vi "ControlCamera.vi"(0 "NumX":i16=640, 1 "StartX":i16=1, 3 "Mode":u16(ring)=4 items=["Exposition guideur"=0, "Guidage"=2, "Piedestal"=3, "Exposition simple"=4, "Mode continu"=5, "Calibration"=8], 4 "ExpTime":dbl, 5 "BinX":i16=1, 6 "N-images(obsolete)":i32, 7 "MaxIm.ICCDCamera":refnum<k7>, 9 "BinY":i16=1, 11 "NumY":i16=480, 12 "StartY":i16=1, 14 "DEC":i16) -> (8 "Done":bool, 10 "ICCDError":errorcluster, 15 "GuiderArrayError":errorcluster)   [LabVIEW 2011]
uses:
  Globals.vi
panel:
  in  "RemoveDark":bool
  out "NumXout":i16=657
  out "NumYout":i16=495
  out "DarkImg":i32[][](array[numeric])
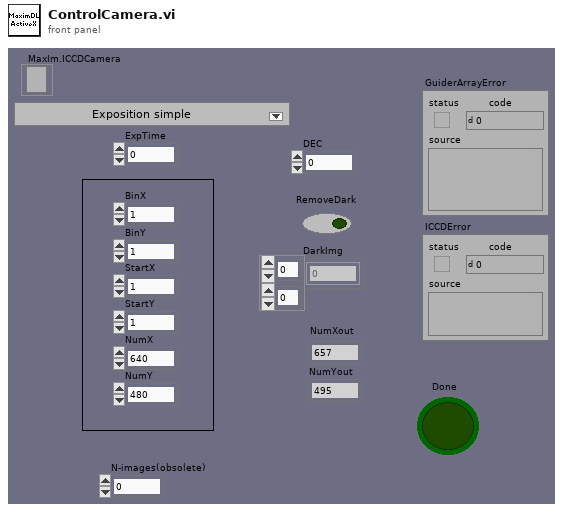
[diagram p1: front panel]
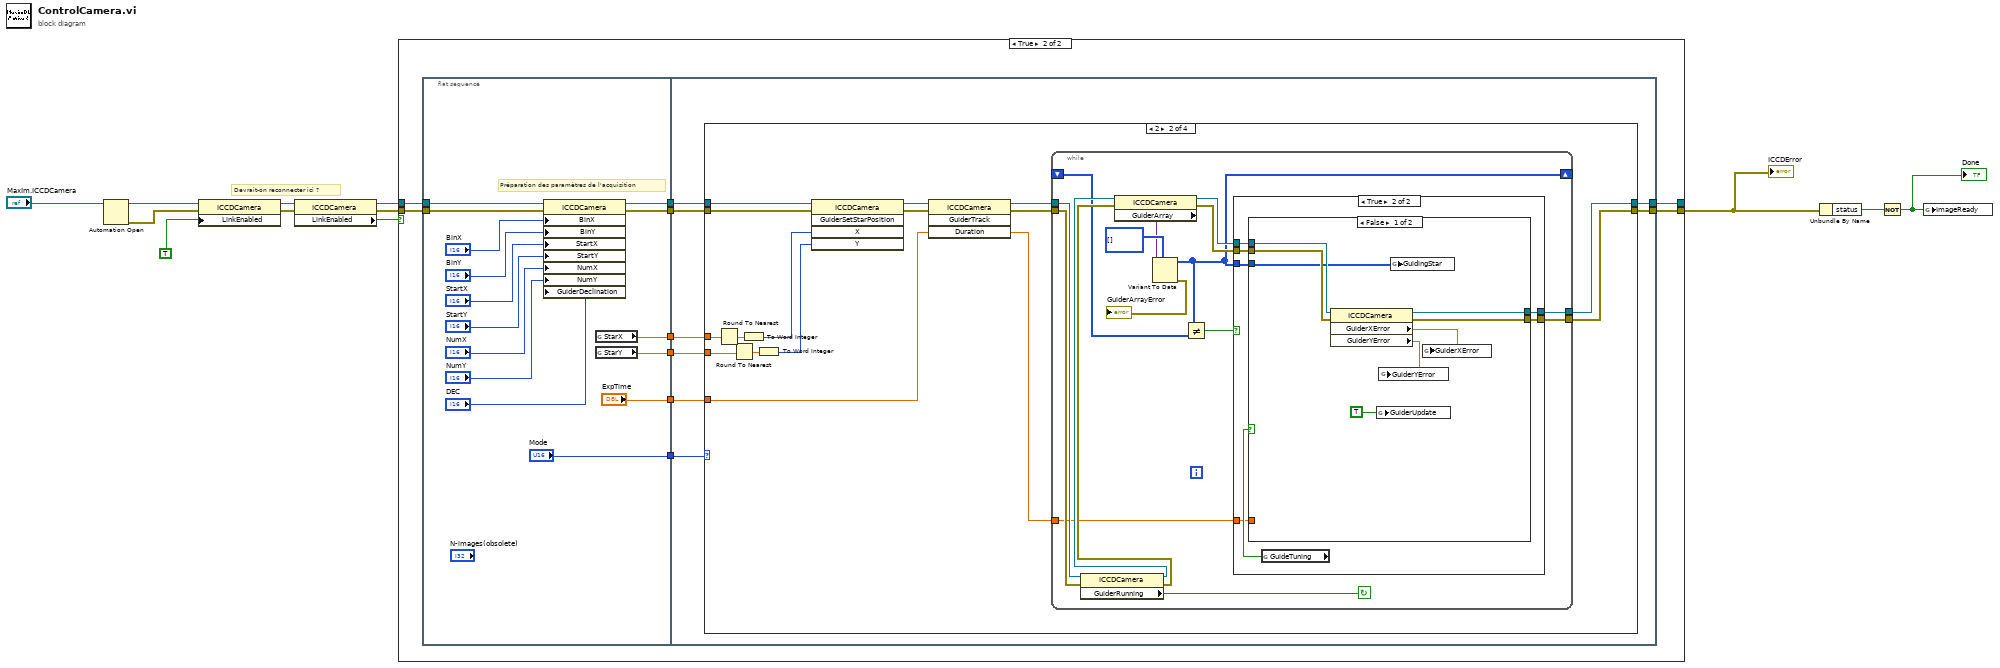
[diagram p0: block diagram]
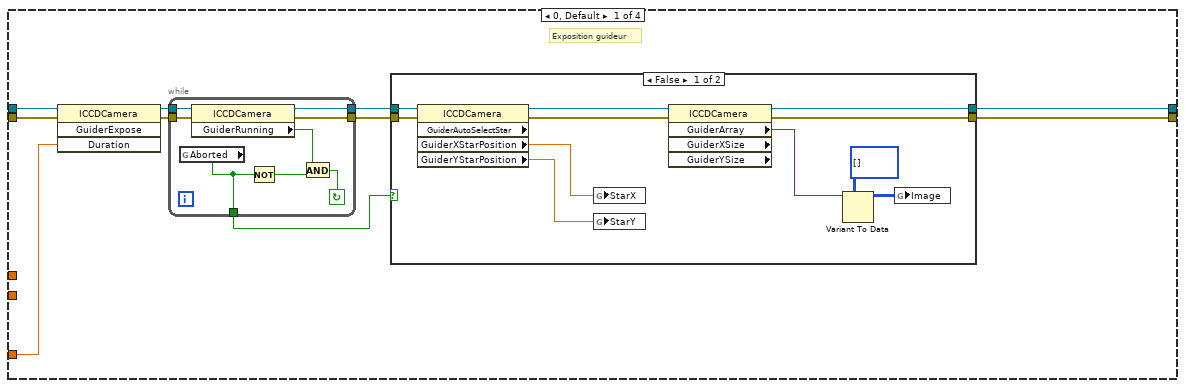
[diagram p3: hidden frame]
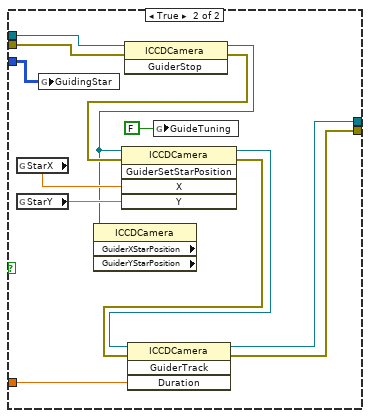
[diagram p6: hidden frame]
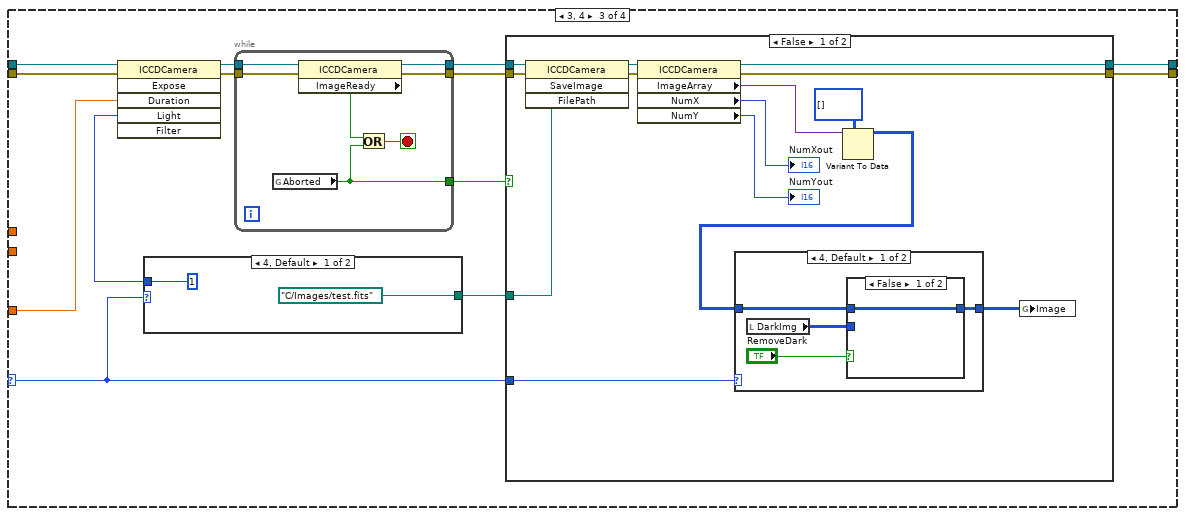
[diagram p7: hidden frame]
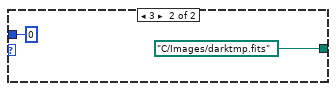
[diagram p8: hidden frame]
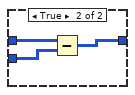
[diagram p9: hidden frame]
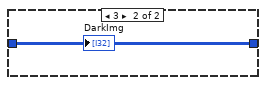
[diagram p10: hidden frame]
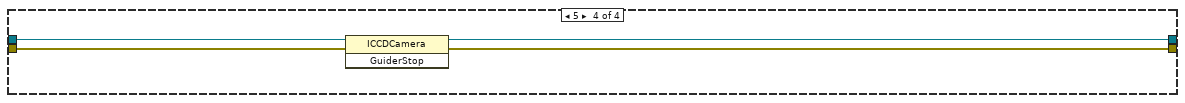
[diagram p12: hidden frame]
diagram:
  # "Devrait-on reconnecter ici ?"
  n1 = Automation Open(Automation Refnum="MaxIm.ICCDCamera") -> (Automation Refnum=w4:refnum<k7>, error out=w3:errorcluster)  [unwired: 3 in]
  n2 = property class="ICCDCamera"(reference=w4, error in=w3, "LinkEnabled"=TRUE) -> (reference out=w6:refnum<k7>, error out=w5:errorcluster)
  n3 = property class="ICCDCamera"(reference=w6, error in=w5) -> (reference out=w10:refnum<k7>, error out=w9:errorcluster, "LinkEnabled"=w11:bool)
  n4 = case shown="True" w11 {
    tunnel: w10 -> [w13 w24]
    tunnel: w9 -> [w14 w22]
    tunnel: [w14 w18] -> w1
    tunnel: [w13 w17] -> _
    frame False {
    }
    frame True {
      n5 = flat-sequence {
        tunnel: w24 -> [w39]
        tunnel: [w38] -> w23
        tunnel: w22 -> [w37]
        tunnel: [w36] -> w21
        tunnel: ["ExpTime"] -> w20
        tunnel: ["Mode"] -> w19
        tunnel: [w27] -> w16
        tunnel: [w26] -> w15
        tunnel: w23 -> [w47]
        tunnel: w21 -> [w46]
        tunnel: w20 -> [w45]
        tunnel: [w44] -> w17
        tunnel: [w43] -> w18
        tunnel: w19 -> [w42]
        tunnel: w16 -> [w41]
        tunnel: w15 -> [w40]
        frame #0 {
          # "Préparation des paramètres de l'acquisition"
          n6 = property class="ICCDCamera"(reference=w39, error in=w37, "BinX"="BinX", "BinY"="BinY", "StartX"="StartX", "StartY"="StartY", "NumX"="NumX", "NumY"="NumY", "GuiderDeclination"="DEC") -> (reference out=w38:refnum<k7>, error out=w36:errorcluster)
          n7 = global read "Globals.vi" "StarX"() -> (w27:sgl)
          n8 = global read "Globals.vi" "StarY"() -> (w26:sgl)
        }
        frame #1 {
          n9 = case shown="2" w42 {
            selector: w42 -> [_ _ w143 _]
            tunnel: w47 -> [w53 w94 w147 w193]
            tunnel: w46 -> [w52 w93 w146 w192]
            tunnel: w45 -> [w51 w84 w148 _]
            tunnel: [w49 w81 w144 w191] -> w44
            tunnel: [w48 w80 w145 w190] -> w43
            tunnel: w41 -> [_ w92 _ _]
            tunnel: w40 -> [_ w88 _ _]
            frame 0, Default {
              # "Exposition guideur"
              n10 = invoke class="ICCDCamera" method="GuiderExpose"(reference=w53, error in=w52, "Duration"=w51) -> (reference out=w57:refnum<k7>, error out=w55:errorcluster)  [unwired: 1 in, 2 out]
              n11 = while {
                tunnel: [w75] -> w54
                tunnel: w55 -> [w76]
                tunnel: [w77] -> w56
                tunnel: w57 -> [w78]
                tunnel: [w71] -> w50
                stop <- w74 continue-if-true
                n12 = global read "Globals.vi" "Aborted"() -> (w71:bool)
                n13 = property class="ICCDCamera"(reference=w78, error in=w76) -> (reference out=w77:refnum<k7>, error out=w75:errorcluster, "GuiderRunning"=w73:bool)
                n14 = Not(x=w71) -> (.not. x?=w72:bool)
                n15 = And(x=w73, y=w72) -> (x .and. y?=w74:bool)
              }
              n16 = case shown="False" w50 {
                tunnel: w56 -> [w68 w70]
                tunnel: w54 -> [w67 w69]
                tunnel: [w59 w70] -> w49
                tunnel: [w58 w69] -> w48
                frame False {
                  n17 = property class="ICCDCamera" props=["GuiderAutoSelectStar", "GuiderXStarPosition", "GuiderYStarPosition"](reference=w68, error in=w67) -> (reference out=w66:refnum<k7>, error out=w60:errorcluster, "GuiderXStarPosition"=w62:sgl, "GuiderYStarPosition"=w61:sgl)  [unwired: 1 out]
                  n18 = global write "Globals.vi" "StarX"(w62) -> ()
                  n19 = global write "Globals.vi" "StarY"(w61) -> ()
                  n20 = property class="ICCDCamera" props=["GuiderArray", "GuiderXSize", "GuiderYSize"](reference=w66, error in=w60) -> (reference out=w59:refnum<k7>, error out=w58:errorcluster, "GuiderArray"=w65:variant)  [unwired: 2 out]
                  n21 = Variant To Data(type=i32[][] [], Variant=w65) -> (data=w63:i32[][])  [unwired: 1 in, 1 out]
                  n22 = global write "Globals.vi" "Image"(w63) -> ()
                }
                frame True {
                }
              }
            }
            frame 2 {
              n23 = Round To Nearest(number=w92) -> (nearest integer value=w91:sgl)
              n24 = Round To Nearest(number=w88) -> (nearest integer value=w89:sgl)
              n25 = To Word Integer(number=w91) -> (16bit integer=w90:i16)
              n26 = To Word Integer(number=w89) -> (16bit integer=w87:i16)
              n27 = invoke class="ICCDCamera" method="GuiderSetStarPosition"(reference=w94, error in=w93, "X"=w90, "Y"=w87) -> (reference out=w86:refnum<k7>, error out=w85:errorcluster)  [unwired: 1 in, 3 out]
              n28 = invoke class="ICCDCamera" method="GuiderTrack"(reference=w86, error in=w85, "Duration"=w84) -> (reference out=w83:refnum<k7>, error out=w82:errorcluster, "Duration"=w79:dbl)  [unwired: 1 in, 1 out]
              n29 = while {
                tunnel: [w108] -> w80
                tunnel: w82 -> [w109]
                tunnel: w83 -> [w110]
                shift-right: [w97] -> _
                shift-left: _ -> [w99]
                tunnel: [w96] -> w81
                tunnel: w79 -> [w95]
                stop <- w107 continue-if-true
                n30 = property class="ICCDCamera"(reference=w110, error in=w109) -> (reference out=w104:refnum<k7>, error out=w103:errorcluster, "GuiderRunning"=w107:bool)
                n31 = property class="ICCDCamera"(reference=w104, error in=w103) -> (reference out=w105:refnum<k7>, error out=w106:errorcluster, "GuiderArray"=w100:variant)
                n32 = Variant To Data(type=i16[][] [], Variant=w100) -> (data=w97:i16[][], error out=→"GuiderArrayError":errorcluster)  [unwired: 1 in]
                n33 = Not Equal?(x=w97, y=w99) -> (x != y?=w101:bool)
                n34 = case shown="True" w101 {
                  tunnel: w106 -> [w112 w117]
                  tunnel: w105 -> [w111 w118]
                  tunnel: [w112 w119] -> w108
                  tunnel: w97 -> [_ w116]
                  tunnel: [w111 w114] -> w96
                  tunnel: w95 -> [_ w113]
                  frame False {
                  }
                  frame True {
                    n35 = global read "Globals.vi" "GuideTuning"() -> (w115:bool)
                    n36 = case shown="False" w115 {
                      tunnel: [w127 w138] -> w119
                      tunnel: w118 -> [w123 w140]
                      tunnel: w117 -> [w122 w139]
                      tunnel: w116 -> [w121 w136]
                      tunnel: [w120 w129] -> w114
                      tunnel: w113 -> [_ w128]
                      frame False {
                        n37 = property class="ICCDCamera"(reference=w123, error in=w122) -> (reference out=w120:refnum<k7>, error out=w127:errorcluster, "GuiderXError"=w126:sgl, "GuiderYError"=w125:sgl)
                        n38 = global write "Globals.vi" "GuiderUpdate"(TRUE ("GuiderUpdate")) -> ()
                        n39 = global write "Globals.vi" "GuiderYError"(w125) -> ()
                        n40 = global write "Globals.vi" "GuidingStar"(w121) -> ()
                        n41 = global write "Globals.vi" "GuiderXError"(w126) -> ()
                      }
                      frame True {
                        n42 = global read "Globals.vi" "StarX"() -> (w132:sgl)
                        n43 = global read "Globals.vi" "StarY"() -> (w131:sgl)
                        n44 = global write "Globals.vi" "GuidingStar"(w136) -> ()
                        n45 = invoke class="ICCDCamera" method="GuiderStop"(reference=w140, error in=w139) -> (reference out=w130:refnum<k7>, error out=w135:errorcluster)  [unwired: 1 in, 1 out]
                        n46 = property class="ICCDCamera" props=["GuiderXStarPosition", "GuiderYStarPosition"](reference=w130) -> ()  [unwired: 1 in, 4 out]
                        n47 = invoke class="ICCDCamera" method="GuiderSetStarPosition"(reference=w130, error in=w135, "X"=w132, "Y"=w131) -> (reference out=w134:refnum<k7>, error out=w133:errorcluster)  [unwired: 1 in, 3 out]
                        n48 = invoke class="ICCDCamera" method="GuiderTrack"(reference=w134, error in=w133, "Duration"=w128) -> (reference out=w129:refnum<k7>, error out=w138:errorcluster)  [unwired: 1 in, 2 out]
                        n49 = global write "Globals.vi" "GuideTuning"(FALSE) -> ()
                      }
                    }
                  }
                }
              }
            }
            frame 3, 4 {
              n50 = case shown="4, Default" w143 {
                tunnel: [path "C:/Images/test.fits" path "C:/Images/darktmp.fits"] -> w142
                tunnel: [i16 1 ("Light") i16 0 ("Light")] -> w141
                frame 4, Default {
                }
                frame 3 {
                }
              }
              n51 = invoke class="ICCDCamera" method="Expose"(reference=w147, error in=w146, "Duration"=w148, "Light"=w141) -> (reference out=w149:refnum<k7>, error out=w151:errorcluster)  [unwired: 2 in, 4 out]
              n52 = while {
                tunnel: [w186] -> w152
                tunnel: w151 -> [w187]
                tunnel: [w188] -> w150
                tunnel: w149 -> [w189]
                tunnel: [w183] -> w153
                stop <- w185 stop-if-true
                n53 = global read "Globals.vi" "Aborted"() -> (w183:bool)
                n54 = property class="ICCDCamera"(reference=w189, error in=w187) -> (reference out=w188:refnum<k7>, error out=w186:errorcluster, "ImageReady"=w184:bool)
                n55 = Or(x=w184, y=w183) -> (x .or. y?=w185:bool)
              }
              n56 = case shown="False" w153 {
                tunnel: w150 -> [w171 w182]
                tunnel: w152 -> [w170 w181]
                tunnel: [w165 w181] -> w145
                tunnel: [w164 w182] -> w144
                tunnel: w143 -> [w162 _]
                tunnel: w142 -> [w163 _]
                frame False {
                  n57 = invoke class="ICCDCamera" method="SaveImage"(reference=w171, error in=w170, "FilePath"=w163) -> (reference out=w169:refnum<k7>, error out=w168:errorcluster)  [unwired: 1 in, 2 out]
                  n58 = property class="ICCDCamera"(reference=w169, error in=w168) -> (reference out=w164:refnum<k7>, error out=w165:errorcluster, "ImageArray"=w160:variant, "NumX"=→"NumXout":i16, "NumY"=→"NumYout":i16)
                  n59 = Variant To Data(type=i32[][] [], Variant=w160) -> (data=w158:i32[][])  [unwired: 1 in, 1 out]
                  n60 = case shown="4, Default" w162 {
                    tunnel: w158 -> [w175 w180]
                    tunnel: [w172 w180] -> w159
                    frame 4, Default {
                      n61 = local read "DarkImg"() -> (w174:i32[][])
                      n62 = case shown="False" "RemoveDark" {
                        tunnel: w175 -> [w176 w179]
                        tunnel: w174 -> [_ w178]
                        tunnel: [w176 w177] -> w172
                        frame False {
                        }
                        frame True {
                          n63 = Subtract(x=w179, y=w178) -> (x-y=w177:i32[][])
                        }
                      }
                    }
                    frame 3 {
                      "DarkImg" <- w180
                    }
                  }
                  n64 = global write "Globals.vi" "Image"(w159) -> ()
                }
                frame True {
                }
              }
            }
            frame 5 {
              n65 = invoke class="ICCDCamera" method="GuiderStop"(reference=w193, error in=w192) -> (reference out=w191:refnum<k7>, error out=w190:errorcluster)  [unwired: 1 in, 1 out]
            }
          }
        }
      }
    }
  }
  "ICCDError" <- w1
  n66 = Unbundle By Name(w1) -> ("status"=w7:bool)
  n67 = Not(x=w7) -> (.not. x?=w8:bool)
  "Done" <- w8
  n68 = global write "Globals.vi" "ImageReady"(w8) -> ()
